vi "_LC Set Method.vi"(5 "Stream#":u8, 6 "Path":path, 7 "Injection Volume":string, 8 "error in (no error)":errorcluster, 9 "Vial Number":string, 10 "Plate Number":string, 11 "Rack Type":string) -> (0 "error out":errorcluster)   [LabVIEW 2012]
uses:
  Type/_LC Command.ctl
  Type/_Log Command.ctl
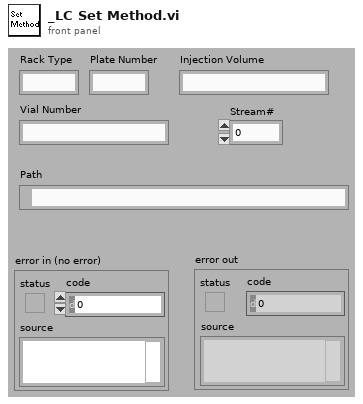
[diagram p1: front panel]
types:
  T1 = cluster{"PlatePosition":u8, "SampleColumn":u8, "TrayType":u8}
  T2 = typedef "_LC Command.ctl" = enum16{"No Command", "Initialize", "Get Configuration", "Get Status", "Get LC Method Contents", "Oven OnOff", "Pump OnOFF", "Rinse Autosampler", "Run Sample", "Set EnvParameters", "Set Method", "Start Equilibration", "Stop Run", "Get LastError", "Clear Error", "Close"}
  T3 = typedef "_Log Command.ctl" = enum16{"No Command", "Open", "Read", "Write", "Close", "Check Size"}
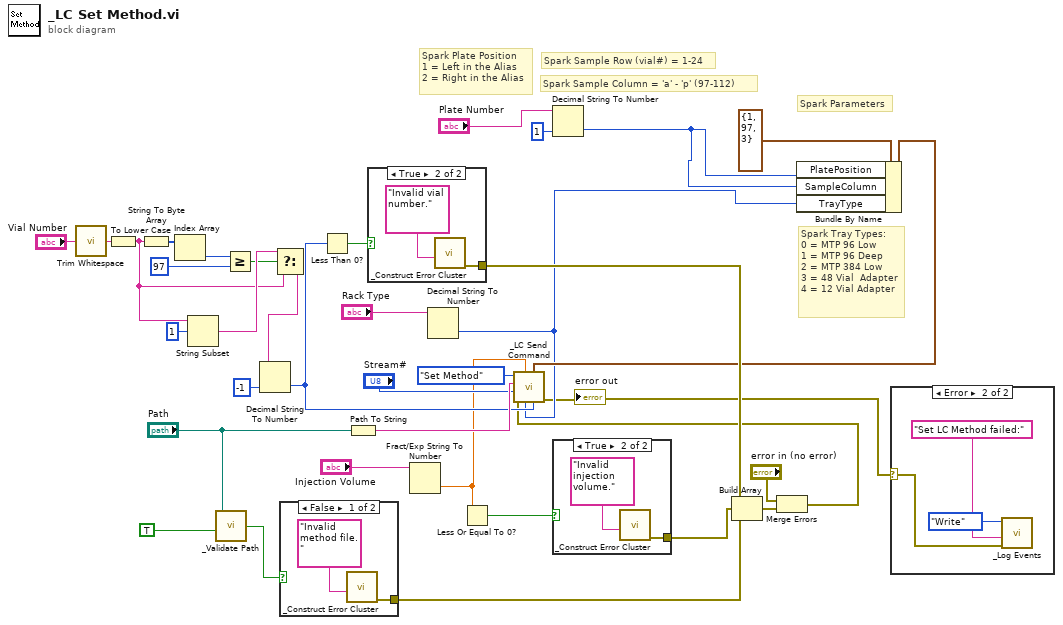
[diagram p0: block diagram]
diagram:
  # "Spark Tray Types:\n0 = MTP 96 Low\n1 = MTP 96 Deep\n2 = MTP 384 Low\n3 = 48 Vial  Adapter\n4 = 12 Vial Adapter"
  # "Spark Parameters"
  # "Spark Sample Column = 'a' - 'p' (97-112)"
  # "Spark Sample Row (vial#) = 1-24"
  # "Spark Plate Position\n1 = Left in the Alias\n2 = Right in the Alias"
  n1 = call <vilib>:"Trim Whitespace.vi"("string"="Vial Number") -> ("trimmed string"=w17:string)  [unwired: 1 in]
  n2 = To Lower Case(string=w17) -> (all lower case string=w12:string)
  n3 = String To Byte Array(string=w12) -> (unsigned byte array=w18:u8[])
  n4 = Index Array(array=w18) -> (element=w6:u8)  [unwired: 1 in]
  n5 = String Subset(string=w12, offset (0)=1) -> (substring=w13:string)  [unwired: 1 in]
  n6 = call "_Validate Path.vi"("Check Exist (F)"=TRUE, "path"="Path") -> ("Valid"=w27:bool)  [unwired: 2 in]
  n7 = Greater Or Equal?(x=w6, y=u8 97) -> (x >= y?=w10:bool)
  n8 = Select(t=w13, s=w10, f=w12) -> (s? t:f=w11:string)
  n9 = Decimal String To Number(string=w11, default (0L)=i16 -1 ("default (0 I32)")) -> (number=w20:i16)  [unwired: 2 out]
  n10 = case shown="False" w27 {
    tunnel: [w38 _] -> w24
    frame False {
      n11 = call "_Construct Error Cluster.vi"("reason"="Invalid method file.") -> ("error out"=w38:errorcluster)  [unwired: 3 in, 3 out]
    }
    frame True {
    }
  }
  n12 = Less Than 0?(x=w20) -> (x < 0?=w30:bool)
  n13 = Path To String(path="Path") -> (string=w32:string)
  n14 = case shown="True" w30 {
    tunnel: [_ w40] -> w26
    frame False {
    }
    frame True {
      n15 = call "_Construct Error Cluster.vi"("reason"="Invalid vial number.") -> ("error out"=w40:errorcluster)  [unwired: 3 in, 3 out]
    }
  }
  n16 = Fract/Exp String To Number(string="Injection Volume") -> (number=w19:dbl)  [unwired: 4 out]
  n17 = Decimal String To Number(string="Rack Type") -> (number=w7:i32)  [unwired: 3 out]
  n18 = Less Or Equal To 0?(x=w19) -> (x <= 0?=w31:bool)
  n19 = Decimal String To Number(string="Plate Number", default (0L)=u8 1 ("default (0 I32)")) -> (number=w2:u8)  [unwired: 2 out]
  n20 = case shown="True" w31 {
    tunnel: [_ w42] -> w25
    frame False {
    }
    frame True {
      n21 = call "_Construct Error Cluster.vi"("reason"="Invalid injection volume.") -> ("error out"=w42:errorcluster)  [unwired: 3 in, 3 out]
    }
  }
  n22 = Build Array(w26, w25, w24) -> (w23:errorcluster[])
  n23 = Merge Errors("error in (no error)", w23) -> (w3:errorcluster)
  n24 = Bundle By Name(cluster=T1 {"PlatePosition"=1, "SampleColumn"=97, "TrayType"=3} ("SparkParameters"), "PlatePosition"=w2, "SampleColumn"=w2, "TrayType"=w7) -> (w8:T1)
  n25 = call "_LC Send Command.vi"("VialNumber"=w20, "SparkParameters"=w8, "RackType"=w7, "InjectionVolume"=w19, "error in"=w3, "Stream#"="Stream#", "Parameter"=w32, "Command"=_LC_Command."Set Method") -> ("error out"=w1:errorcluster)  [unwired: 2 in, 1 out]
  "error out" <- w1
  n26 = case shown="Error" w1 {
    selector: w1 -> [_ w43]
    frame No Error {
    }
    frame Error {
      n27 = call "_Log Events.vi"("error in (no error)"=w43, "Event"="Set LC Method failed:", "Log Command"=_Log_Command."Write") -> ()  [unwired: 1 in, 5 out]
    }
  }
